vi "Library Path.vi"() -> (0 "Library Path":path=path "C:/LQWidgets/LQWidgets.dll")   [LabVIEW 2013, in "Template.lvlib" / "LQWidgetEngine.lvclass"]
uses:
  LQWidgetEngine.lvclass
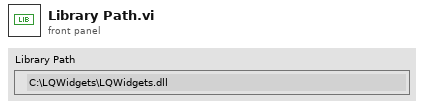
[diagram p1: front panel]
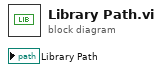
[diagram p0: block diagram]
diagram:
